vi "DBL Read from Buffer.vi"(8 "error in (no error)":errorcluster, 9 "Length":i32, 10 "Start Index":i32, 11 "DBL Waveform Buffer in":refnum<class "DBL Waveform Buffer.lvclass">) -> (0 "error out":errorcluster, 2 "Data":dbl[](array[numeric]), 3 "DBL Waveform Buffer out":refnum<class "DBL Waveform Buffer.lvclass">)   [LabVIEW 2012, in "Waveform Data Logger Engine.lvlib" / "DBL Waveform Buffer.lvclass"]
uses:
  DBL Waveform Buffer.lvclass
  Waveform Buffer/Waveform Buffer.lvclass/Waveform Buffer.ctl
  DBL Waveform Buffer.lvclass/DBL Waveform Buffer.ctl
  Waveform Buffer/Waveform Buffer.lvclass
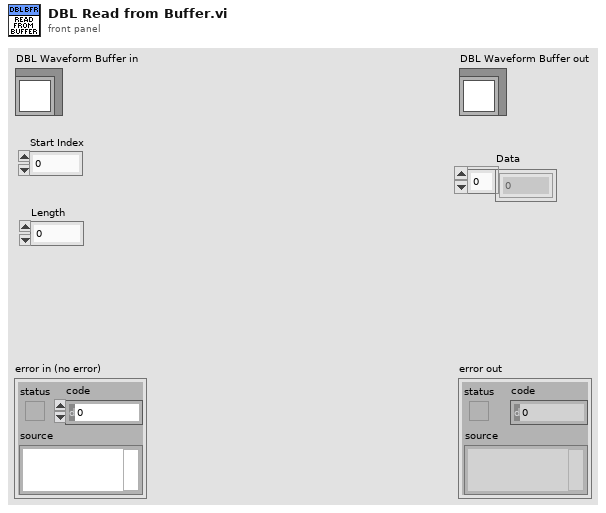
[diagram p1: front panel]
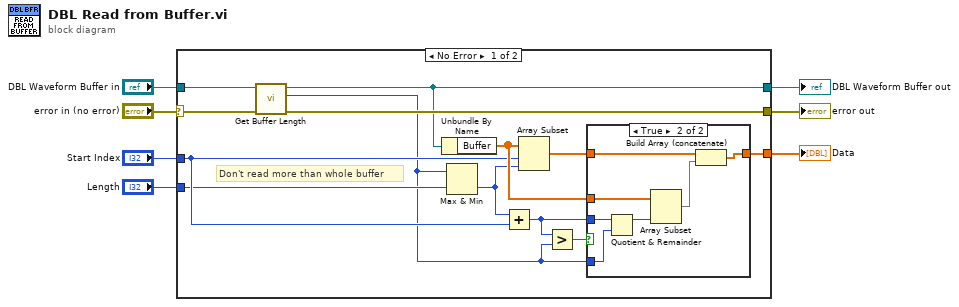
[diagram p0: block diagram]
diagram:
  n1 = case shown="No Error" "error in (no error)" {
    selector: "error in (no error)" -> [w11 w30]
    tunnel: [w10 w30] -> w6
    tunnel: [w9 w29] -> w4
    tunnel: "DBL Waveform Buffer in" -> [w12 w29]
    tunnel: "Start Index" -> [w17 _]
    tunnel: "Length" -> [w16 _]
    tunnel: [w19 _] -> w1
    frame No Error {
      # "Don't read more than whole buffer"
      n2 = call "Get Buffer Length.vi"("error in (no error)"=w11, "Waveform Buffer in"=w12) -> ("error out"=w10:errorcluster, "Length"=w8:i32, "Waveform Buffer out"=w9:refnum<class "DBL Waveform Buffer.lvclass">)  [unwired: 7 in]
      n3 = Unbundle By Name(w9) -> ("Buffer"=w18:dbl[])
      n4 = Max & Min(x=w8, y=w16) -> (min(x,y)=w15:i32)  [unwired: 1 out]
      n5 = Add(x=w15, y=w17) -> (x+y=w14:i32)
      n6 = Array Subset(array=w18, index=w17, length=w15) -> (w13:dbl[])
      n7 = Greater?(x=w14, y=w8) -> (0:w20:bool)
      n8 = case shown="True" w20 {
        tunnel: w13 -> [w21 w28]
        tunnel: [w21 w26] -> w19
        tunnel: w18 -> [_ w25]
        tunnel: w14 -> [_ w24]
        tunnel: w8 -> [_ w23]
        frame False {
        }
        frame True {
          n9 = Quotient & Remainder(x=w24, y=w23) -> (x-y*floor(x/y)=w22:i32)  [unwired: 1 out]
          n10 = Array Subset(array=w25, length=w22) -> (w27:dbl[])  [unwired: 1 in]
          n11 = Build Array (concatenate)(w28, w27) -> (w26:dbl[])
        }
      }
    }
    frame Error {
    }
  }
  "error out" <- w6
  "DBL Waveform Buffer out" <- w4
  "Data" <- w1
